vi "NXT_HINDBRAIN Scale Motor Command.vi"(1 "command":i32, 2 "min":u16, 3 "mid":u16, 4 "max":u16) -> (0 "converted":u16)   [LabVIEW 2012, in "Tugboat.lvrbt"]
uses:
  Tugboat.lvrbt
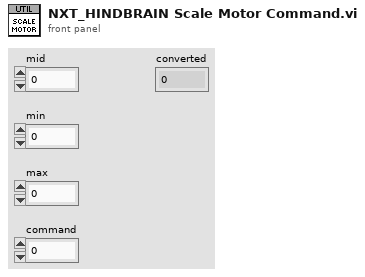
[diagram p1: front panel]
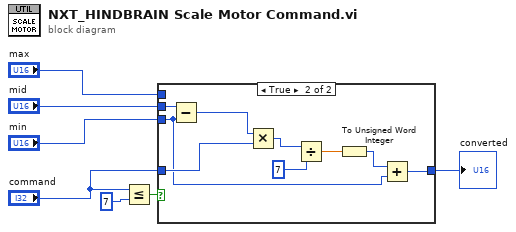
[diagram p0: block diagram]
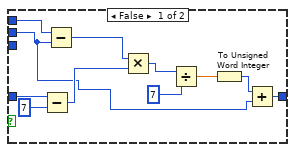
[diagram p2: hidden frame]
diagram:
  n1 = Less Or Equal?(x="command", y=7) -> (x <= y?=w1:bool)
  n2 = case shown="True" w1 {
    tunnel: "command" -> [w13 w25]
    tunnel: "min" -> [_ w19]
    tunnel: "max" -> [w14 _]
    tunnel: "mid" -> [w8 w27]
    tunnel: [w10 w21] -> w7
    frame False {
      n3 = Subtract(x=w13, y=7) -> (x-y=w11:i32)
      n4 = Subtract(x=w14, y=w8) -> (x-y=w15:u16)
      n5 = Multiply(x=w15, y=w11) -> (x*y=w16:i32)
      n6 = Divide(x=w16, y=7) -> (x/y=w18:dbl)
      n7 = To Unsigned Word Integer(number=w18) -> (unsigned 16bit integer=w9:u16)
      n8 = Add(x=w9, y=w8) -> (x+y=w10:u16)
    }
    frame True {
      n9 = Subtract(x=w27, y=w19) -> (x-y=w26:u16)
      n10 = Multiply(x=w26, y=w25) -> (x*y=w24:i32)
      n11 = Divide(x=w24, y=7) -> (x/y=w22:dbl)
      n12 = To Unsigned Word Integer(number=w22) -> (unsigned 16bit integer=w20:u16)
      n13 = Add(x=w20, y=w19) -> (x+y=w21:u16)
    }
  }
  "converted" <- w7
